vi "MeasAction.vi"(8 "error in (no error)":errorcluster caption="entrée d'erreur (pas d'erreur)", 9 "CurvePointIndex":i32, 10 "AllPointIndex":i32, 11 "InstrClassIn":refnum<class "HeFlowMeter.lvclass"> caption="DNL_LabVIEW Object in") -> (0 "error out":errorcluster caption="sortie d'erreur", 2 "MeasDatOut":dbl[](array[numeric]), 3 "InstrClassOut":refnum<class "HeFlowMeter.lvclass"> caption="DNL_LabVIEW Object out")   [LabVIEW 2019, in "HeFlowMeter.lvclass"]
uses:
  HeFlowMeter.lvclass
  C:/Programmes Labview/LabscanV1A/DevicesClass/BaseDevice/BaseDevice.lvclass
  HeFlowMeter.lvclass/HeFlowMeter.ctl
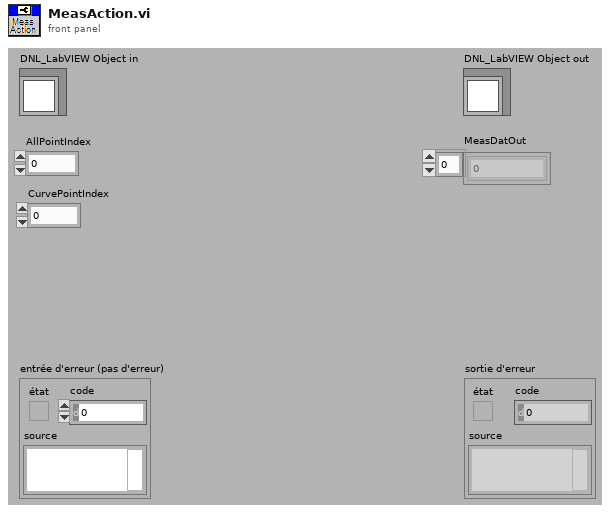
[diagram p1: front panel]
types:
  T1 = typedef "HeFlowMeter.lvclass/HeFlowMeter_Func.ctl" = enum16{"ReadFlow (m3h-1)"}
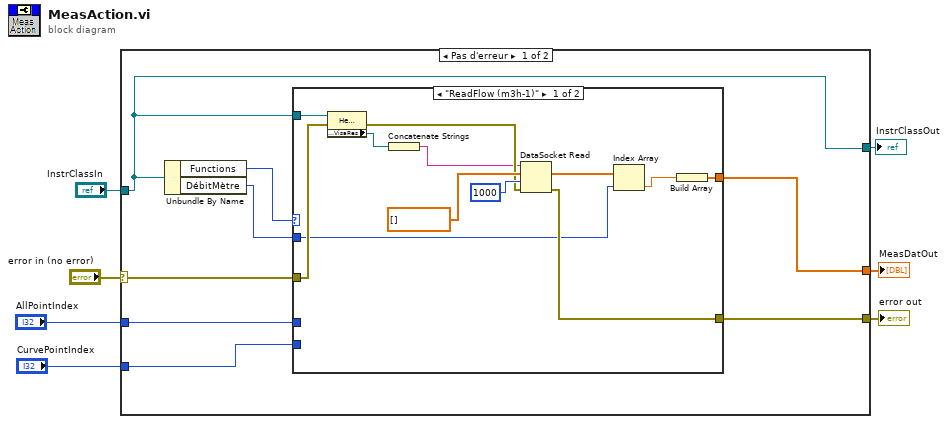
[diagram p0: block diagram]
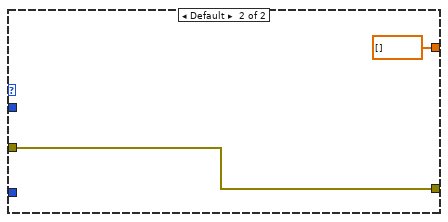
[diagram p2: hidden frame]
diagram:
  n1 = case shown="Pas d'erreur" "error in (no error)" {
    selector: "error in (no error)" -> [w11 w30]
    tunnel: "InstrClassIn" -> [w9 w31]
    tunnel: [w9 w31] -> w5
    tunnel: "AllPointIndex" -> [w15 _]
    tunnel: [w14 w30] -> w3
    tunnel: [w13 _] -> w2
    tunnel: "CurvePointIndex" -> [w10 _]
    frame No Error {
      n2 = Unbundle By Name(w9) -> ("Functions"=w12:T1, "DébitMètre"=w8:u16)
      n3 = case shown="\"ReadFlow (m3h-1)\"" w12 {
        tunnel: w15 -> [_ _]
        tunnel: [w21 w28] -> w14
        tunnel: [w23 dbl[] [] ("Outputs")] -> w13
        tunnel: w11 -> [w20 w28]
        tunnel: w10 -> [_ _]
        tunnel: w9 -> [w22 _]
        tunnel: w8 -> [w16 _]
        frame "ReadFlow (m3h-1)" {
          n4 = property class="HeFlowMeter.lvclass"(reference=w22, error in=w20) -> (error out=w19:errorcluster, "Accessor:VisaRes"=w18:refnum<visa-resource-name>)  [unwired: 1 out]
          n5 = Concatenate Strings(w18) -> (w17:string)
          n6 = DataSocket Read(8:w19, 9:1000 ("timeout en ms (10000)"), 10:dbl[] [], 11:w17) -> (0:w21:errorcluster, 2:w25:dbl[])  [unwired: 6 out]
          n7 = Index Array(array=w25, index=w16) -> (element=w24:dbl)
          n8 = Build Array(w24) -> (w23:dbl[])
        }
        frame Default {
        }
      }
    }
    frame Error {
    }
  }
  "error out" <- w3
  "InstrClassOut" <- w5
  "MeasDatOut" <- w2
